vi "Config Template.vi"() -> (1 "Template Image":T1(plugin-control), 2 "Template Mask":T1(plugin-control), 3 "Cancelado?":bool=TRUE, 4 "error out":errorcluster)   [LabVIEW 2020]
uses:
  Type Defs/Config Template Events.ctl
  <vilib>/vision/Image Controls.llb/IMAQ Image.ctl
  <vilib>/vision/NI_Vision_Development_Module.lvlib
panel:
  in  "Cortar Imagem":bool
  in  "Sair":bool
  in  "Montar Máscara":bool
  in  "Carregar Imagem":bool
  in  "OK Button":bool
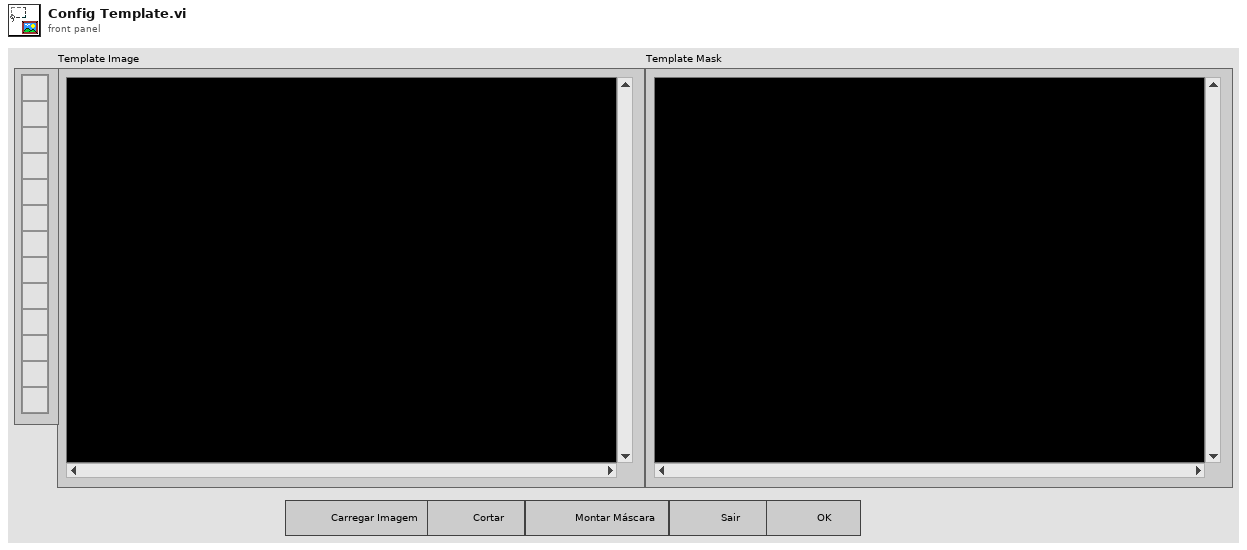
[diagram p1: front panel]
types:
  T1 = typedef "IMAQ Image.ctl" = refnum<image>
  T2 = typedef "Config Template Events.ctl" = enum16{"Aguardar", "Inicializar", "Selecionar Imagem", "Salvar Template", "Cortar", "Montar máscara", "Sair"}
  T3 = cluster{"Global Rectangle":i32[], "Contours":cluster{"Contour Type":u32, "ROI Type":u32, "Points":i32[]}[]}
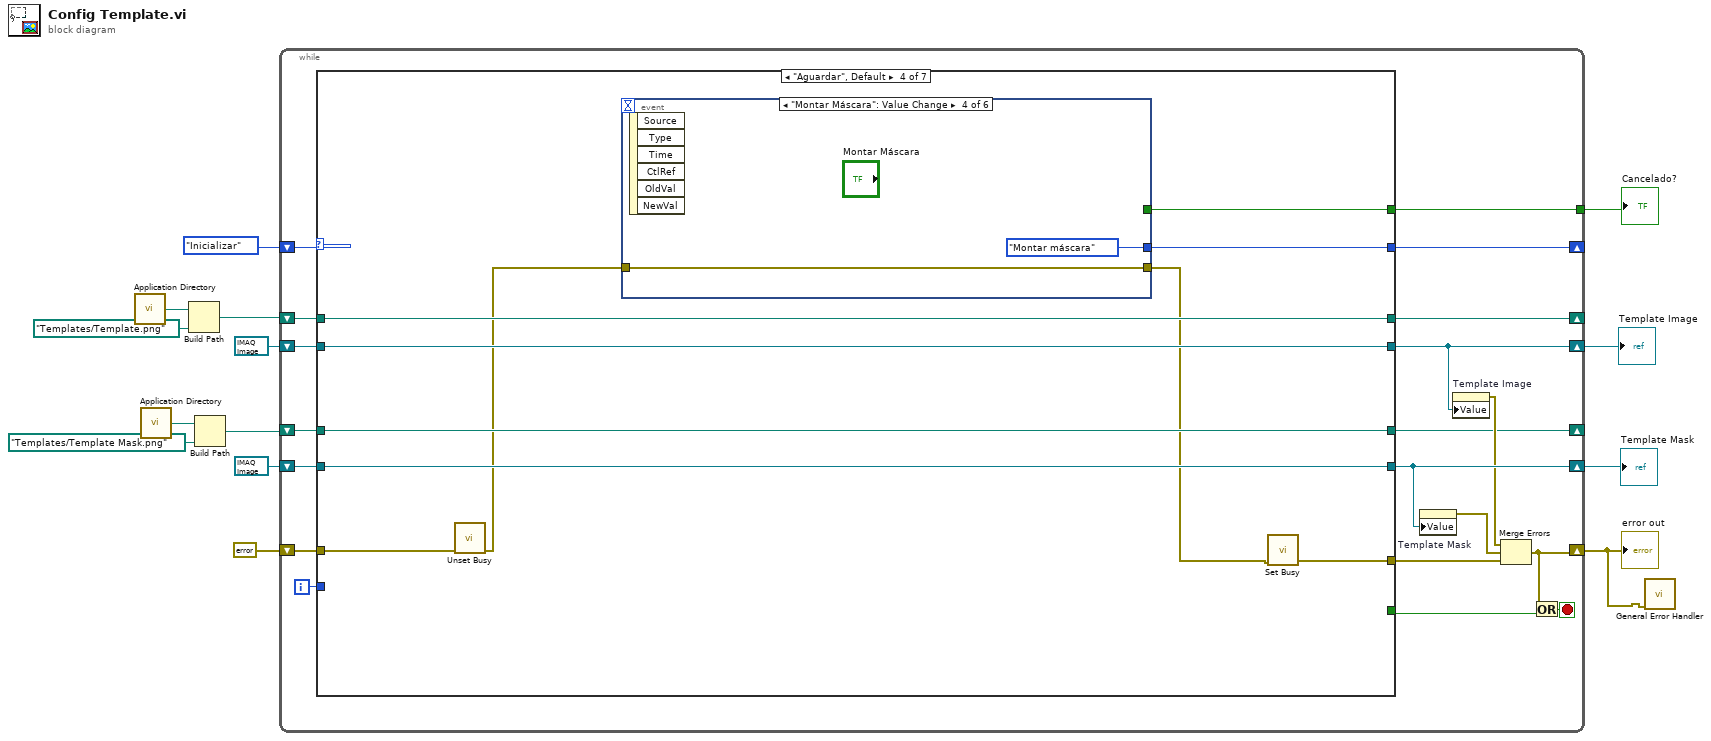
[diagram p0: block diagram]
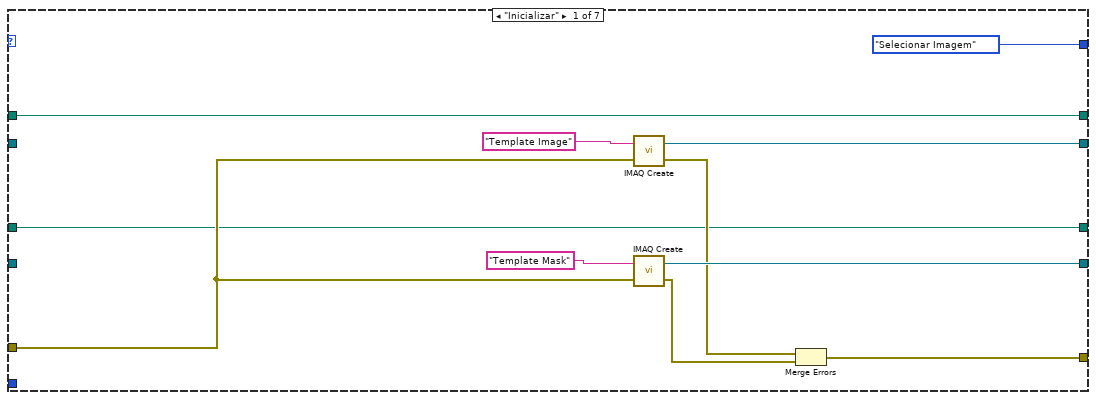
[diagram p2: hidden frame]
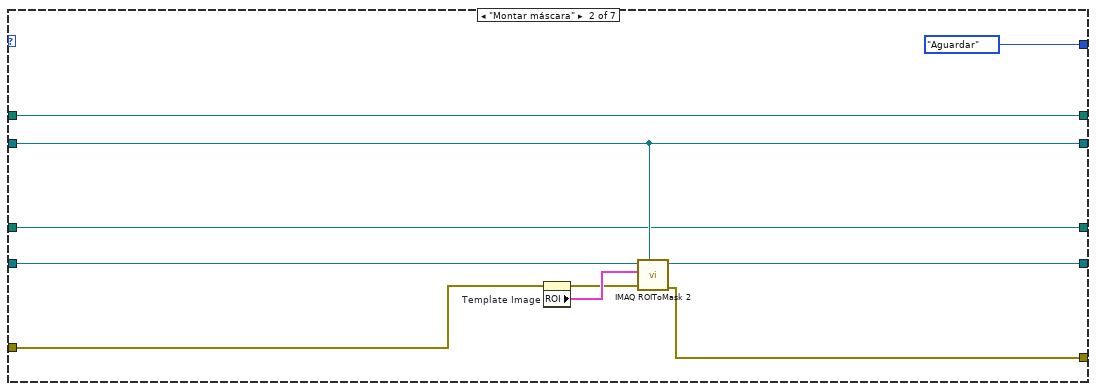
[diagram p3: hidden frame]
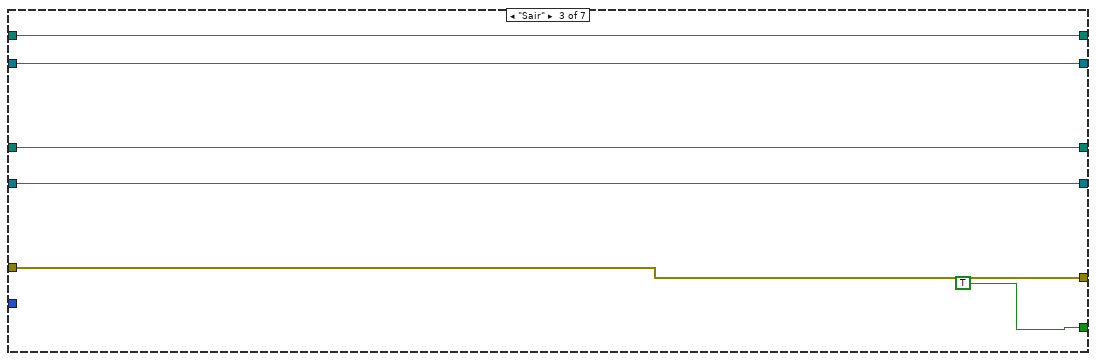
[diagram p4: hidden frame]
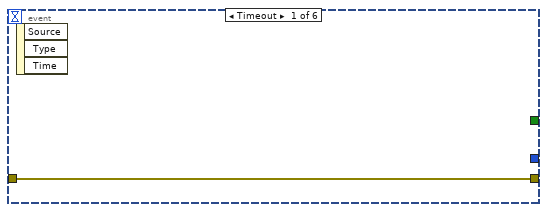
[diagram p5: hidden frame]
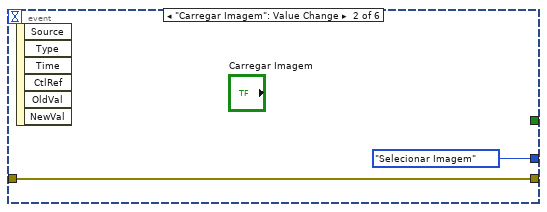
[diagram p6: hidden frame]
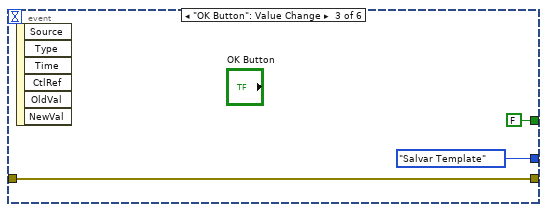
[diagram p7: hidden frame]
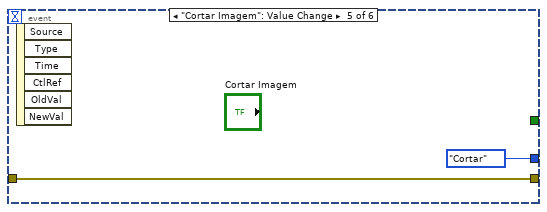
[diagram p8: hidden frame]
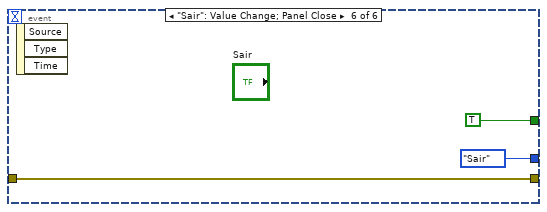
[diagram p9: hidden frame]
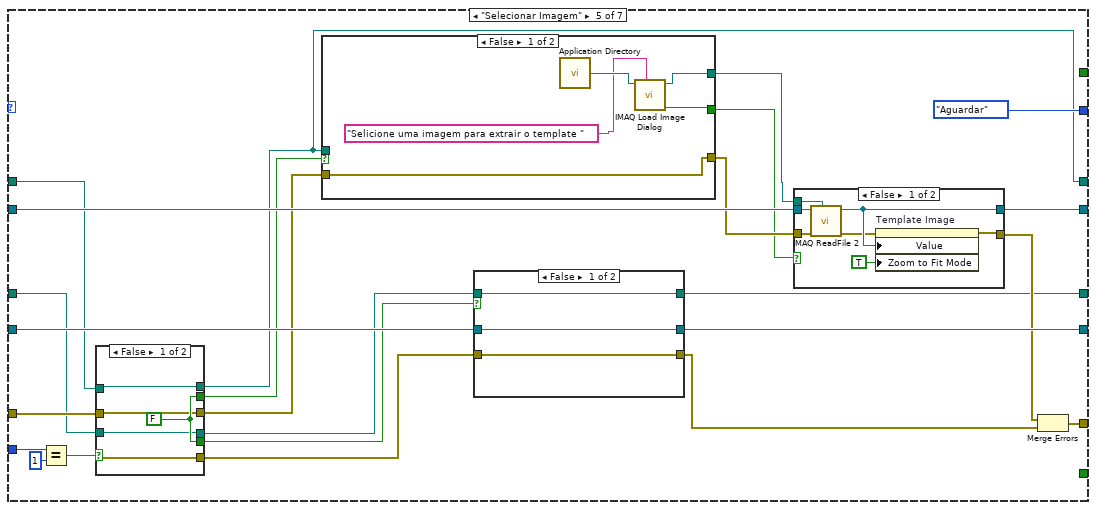
[diagram p10: hidden frame]
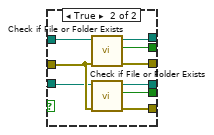
[diagram p11: hidden frame]
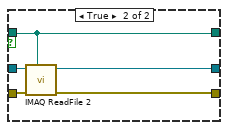
[diagram p12: hidden frame]
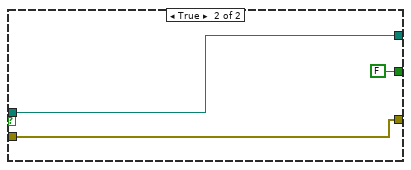
[diagram p13: hidden frame]
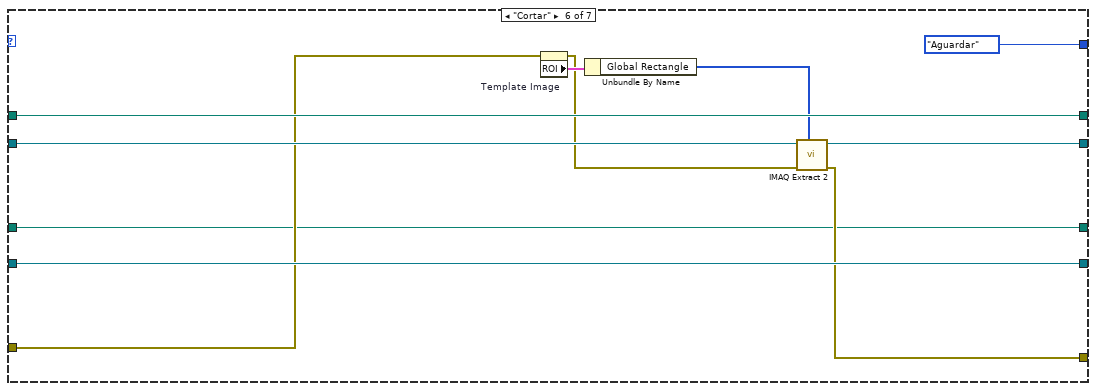
[diagram p15: hidden frame]
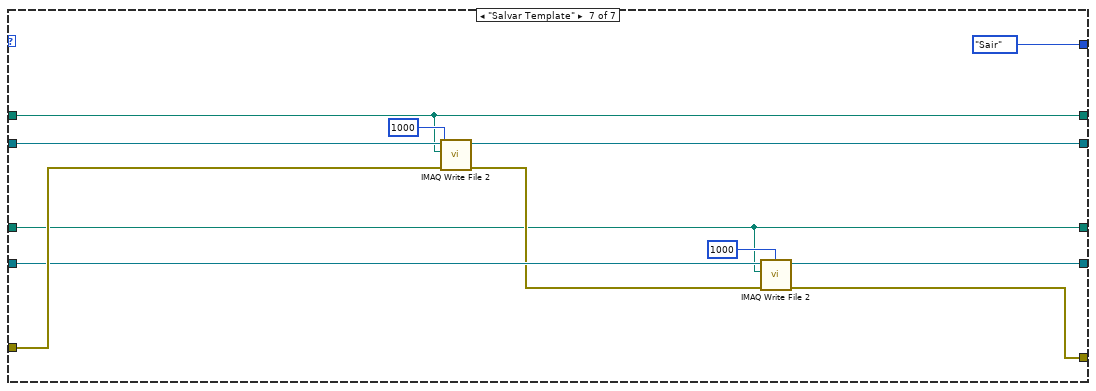
[diagram p16: hidden frame]
diagram:
  n1 = call <vilib>:"Application Directory.vi"() -> ("Application Directory"=w7:path)
  n2 = call <vilib>:"Application Directory.vi"() -> ("Application Directory"=w4:path)
  n3 = Build Path(base path=w7, name or relative path=path "Templates/Template.png") -> (appended path=w5:path)
  n4 = Build Path(base path=w4, name or relative path=path "Templates/Template Mask.png") -> (appended path=w2:path)
  n5 = while {
    shift-right: [w32] -> _
    shift-left: w5 -> [w25]
    shift-right: [w31] -> _
    shift-left: Config_Template_Events."Inicializar" -> [w33]
    shift-right: [w24] -> w13
    shift-left: T1 refnum ("Image Out (duplicate)") -> [w30]
    shift-right: [w23] -> w12
    shift-left: T1 refnum ("Image Out (duplicate)") -> [w28]
    shift-right: [w22] -> w1
    shift-left: errorcluster {"status"=FALSE, "code"=0, "source"=""} ("error Constant") -> [w29]
    tunnel: [w18] -> w11
    shift-right: [w17] -> _
    shift-left: w2 -> [w16]
    i -> [w15]
    stop <- w26 stop-if-true
    n6 = case shown="\"Aguardar\", Default" w33 {
      tunnel: [w35 w47 w56 w66 w84 w155 w158] -> w32
      tunnel: [Config_Template_Events."Selecionar Imagem" Config_Template_Events."Aguardar" _ w70 Config_Template_Events."Aguardar" Config_Template_Events."Aguardar" Config_Template_Events."Sair"] -> w31
      tunnel: [w41 w52 w59 w69 w103 w153 w164] -> w24
      tunnel: [w40 w53 w58 w68 w101 w156 w162] -> w23
      tunnel: w30 -> [_ w52 w59 w69 w105 w154 w167]
      tunnel: [w36 w50 w57 w62 w98 w148 w160] -> w21
      tunnel: w29 -> [w39 w48 w57 w64 w92 w152 w165]
      tunnel: w28 -> [_ w51 w58 w68 w102 w156 w163]
      tunnel: [_ _ TRUE _ _ _ _] -> w27
      tunnel: w25 -> [w35 w47 w56 w66 w86 w155 w158]
      tunnel: [_ _ _ w67 _ _ _] -> w18
      tunnel: [w34 w45 w55 w65 w95 w146 w157] -> w17
      tunnel: w16 -> [w34 w45 w55 w65 w85 w146 w157]
      tunnel: w15 -> [_ _ _ _ w89 _ _]
      frame "Inicializar" {
        n7 = call "IMAQ Create"("Image Name"="Template Image", "error in (no error)"=w39) -> ("New Image"=w41:T1, "error out"=w38:errorcluster)  [unwired: 3 in]
        n8 = call "IMAQ Create"("Image Name"="Template Mask", "error in (no error)"=w39) -> ("New Image"=w40:T1, "error out"=w37:errorcluster)  [unwired: 3 in]
        n9 = Merge Errors(w38, w37) -> (w36:errorcluster)
      }
      frame "Montar máscara" {
        n10 = property on="Template Image" class="ImageControl"(error in=w48) -> (error out=w49:errorcluster, "ROI"=w54:T3)  [unwired: 1 in, 1 out]
        n11 = call "IMAQ ROIToMask 2"("Image Model"=w52, "error in (no error)"=w49, "ROI Descriptor"=w54, "Image"=w51) -> ("error out"=w50:errorcluster, "Image Out"=w53:T1)  [unwired: 5 in, 1 out]
      }
      frame "Sair" {
      }
      frame "Aguardar", Default {
        n12 = call <vilib>:"Unset Busy.vi"("error in (no error)"=w64) -> ("error out"=w63:errorcluster)  [unwired: 10 in]
        n13 = event shown="[3] \"Montar Máscara\": Value Change" {
          selector: _ -> [_ _ _ _ _ _]
          dyn-events: _ -> [_ _ _ _ _ _]
          timeout: _ -> [_ _ _ _ _ _]
          tunnel: [_ Config_Template_Events."Selecionar Imagem" Config_Template_Events."Salvar Template" Config_Template_Events."Montar máscara" Config_Template_Events."Cortar" Config_Template_Events."Sair"] -> w70
          tunnel: [_ _ FALSE _ _ TRUE] -> w67
          tunnel: w63 -> [w71 w72 w74 w77 w79 w81]
          tunnel: [w71 w72 w74 w77 w79 w81] -> w61
          event Timeout {
            n14 = event-data() -> ()  [unwired: 1 in, 3 out]
          }
          event "Carregar Imagem": Value Change {
            n15 = event-data() -> ()  [unwired: 1 in, 6 out]
          }
          event "OK Button": Value Change {
            n16 = event-data() -> ()  [unwired: 1 in, 6 out]
          }
          event "Montar Máscara": Value Change {
            n17 = event-data() -> ()  [unwired: 1 in, 6 out]
          }
          event "Cortar Imagem": Value Change {
            n18 = event-data() -> ()  [unwired: 1 in, 6 out]
          }
          event "Sair": Value Change; Panel Close {
            n19 = event-data() -> ()  [unwired: 1 in, 3 out]
          }
        }
        n20 = call <vilib>:"Set Busy.vi"("error in (no error)"=w61) -> ("error out"=w62:errorcluster)  [unwired: 9 in, 1 out]
      }
      frame "Selecionar Imagem" {
        n21 = Equal?(x=w89, y=1) -> (x = y?=w87:bool)
        n22 = case shown="False" w87 {
          tunnel: [w108 w120] -> w100
          tunnel: [w111 w119] -> w99
          tunnel: [w109 w118] -> w84
          tunnel: [w111 w117] -> w93
          tunnel: w92 -> [w110 w116]
          tunnel: [w110 w115] -> w91
          tunnel: [w110 w114] -> w90
          tunnel: w86 -> [w109 w113]
          tunnel: w85 -> [w108 w112]
          frame False {
            w111 = FALSE ("file or folder exists?")
          }
          frame True {
            n23 = call <vilib>:"Check if File or Folder Exists.vi"("error in (no error)"=w116, "path"=w113) -> ("error out"=w114:errorcluster, "file or folder exists?"=w117:bool, "dup path"=w118:path)  [unwired: 7 in]
            n24 = call <vilib>:"Check if File or Folder Exists.vi"("error in (no error)"=w116, "path"=w112) -> ("error out"=w115:errorcluster, "file or folder exists?"=w119:bool, "dup path"=w120:path)  [unwired: 7 in]
          }
        }
        n25 = case shown="False" w93 {
          tunnel: [w132 w135] -> w106
          tunnel: [w129 w134] -> w104
          tunnel: [w131 FALSE ("cancelled")] -> w94
          tunnel: w84 -> [_ w135]
          tunnel: w90 -> [w129 w134]
          frame False {
            n26 = call <vilib>:"Application Directory.vi"() -> ("Application Directory"=w133:path)
            n27 = call "IMAQ Load Image Dialog"("Prompt"="Selicione uma imagem para extrair o template " ("prompt"), "Start Path"=w133) -> ("Cancelled?"=w131:bool, "Path"=w132:path)  [unwired: 7 in, 1 out]
          }
          frame True {
          }
        }
        n28 = case shown="False" w99 {
          tunnel: w100 -> [w122 w125]
          tunnel: w102 -> [w123 w128]
          tunnel: [w123 w127] -> w101
          tunnel: [w121 w126] -> w97
          tunnel: [w122 w125] -> w95
          tunnel: w91 -> [w121 w124]
          frame False {
          }
          frame True {
            n29 = call "IMAQ ReadFile 2"("File Path"=w125, "error in (no error)"=w124, "Image"=w128) -> ("error out"=w126:errorcluster, "Image Out"=w127:T1)  [unwired: 4 in, 3 out]
          }
        }
        n30 = case shown="False" w94 {
          tunnel: w106 -> [w143 _]
          tunnel: w105 -> [w142 w145]
          tunnel: w104 -> [w141 w144]
          tunnel: [w140 w145] -> w103
          tunnel: [w137 w144] -> w96
          frame False {
            n31 = call "IMAQ ReadFile 2"("File Path"=w143, "error in (no error)"=w141, "Image"=w142) -> ("error out"=w138:errorcluster, "Image Out"=w140:T1)  [unwired: 4 in, 3 out]
            n32 = property on="Template Image" class="ImageControl"(error in=w138, "Value"=w140, "Zoom to Fit Mode"=TRUE) -> (error out=w137:errorcluster)  [unwired: 1 in, 1 out]
          }
          frame True {
          }
        }
        n33 = Merge Errors(w96, w97) -> (w98:errorcluster)
      }
      frame "Cortar" {
        n34 = property on="Template Image" class="ImageControl"(error in=w152) -> (error out=w149:errorcluster, "ROI"=w151:T3)  [unwired: 1 in, 1 out]
        n35 = Unbundle By Name(w151) -> ("Global Rectangle"=w150:i32[])
        n36 = call "IMAQ Extract 2"("Optional Rectangle"=w150, "error in (no error)"=w149, "Image Src"=w154) -> ("error out"=w148:errorcluster, "Image Dst Out"=w153:T1)  [unwired: 7 in]
      }
      frame "Salvar Template" {
        n37 = call-poly "IMAQ Write File 2"("error in (no error)"=w165, "Image Quality"=u32 1000, "File Path"=w158, "Image"=w167) -> ("error out"=w161:errorcluster, "Image Out (duplicate)"=w164:T1)  [unwired: 6 in]
        n38 = call-poly "IMAQ Write File 2"("error in (no error)"=w161, "Image Quality"=u32 1000, "File Path"=w157, "Image"=w163) -> ("error out"=w160:errorcluster, "Image Out (duplicate)"=w162:T1)  [unwired: 6 in]
      }
    }
    n39 = property on="Template Mask" class="ImageControl"("Value"=w23) -> (error out=w20:errorcluster)  [unwired: 2 in, 1 out]
    n40 = property on="Template Image" class="ImageControl"("Value"=w24) -> (error out=w19:errorcluster)  [unwired: 2 in, 1 out]
    n41 = Merge Errors(w19, w20, w21) -> (w22:errorcluster)
    n42 = Or(x=w22, y=w27) -> (x .or. y?=w26:bool)
  }
  "Template Image" <- w13
  "Template Mask" <- w12
  "error out" <- w1
  "Cancelado?" <- w11
  n43 = call <vilib>:"General Error Handler.vi"("error in (no error)"=w1) -> ()  [unwired: 10 in, 5 out]
